vi "Receive Read Data Parse.vi"(8 "error in (no error)":errorcluster, 10 "Specified Num in":u8=1, 11 "Received Read Data":string) -> (0 "error out":errorcluster, 1 "CRC Check?":bool, 2 "Data":i32[](array[numeric]), 3 "Received Read Data":u8[](array[numeric]) format="%.0x")   [LabVIEW 2014, in "ALPHA5 RS485.lvlib"]
uses:
  ALPHA5 RS485.lvlib
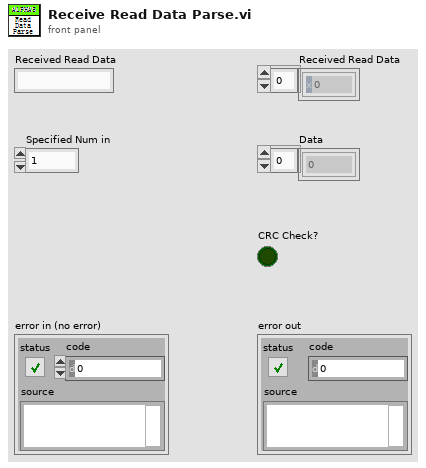
[diagram p1: front panel]
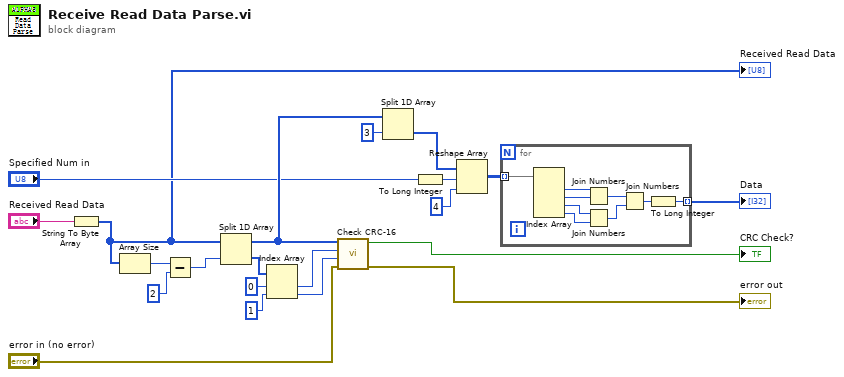
[diagram p0: block diagram]
diagram:
  n1 = String To Byte Array(string="Received Read Data") -> (unsigned byte array=w4:u8[])
  "Received Read Data" <- w4
  n2 = Array Size(array=w4) -> (size(s)=w20:i32)
  n3 = Subtract(x=w20, y=2 ("index")) -> (x-y=w18:i32)
  n4 = Split 1D Array(array=w4, index=w18) -> (first subarray=w12:u8[], second subarray=w17:u8[])
  n5 = Index Array(array=w17, index #1=0 ("index"), index #2=1 ("index")) -> (element #1=w14:u8, element #2=w13:u8)
  n6 = call "Check CRC-16.vi"("error in (no error)"="error in (no error)", "CRC-16-H"=w13, "CRC-16-L"=w14, "Data In"=w12) -> ("error out"=→"error out":errorcluster, "Check Result"=→"CRC Check?":bool)  [unwired: 6 in]
  n7 = Split 1D Array(array=w12, index=3) -> (second subarray=w10:u8[])  [unwired: 1 out]
  n8 = To Long Integer(number="Specified Num in") -> (32bit integer=w9:i32)
  n9 = Reshape Array(w10, w9, 4 ("dimension size")) -> (w7:u8[][])
  n10 = for {
    tunnel: w7 -> [w28] mode=indexing
    tunnel: [w22] -> w6 mode=indexing
    n11 = Index Array(array=w28) -> (element #1=w27:u8, element #2=w26:u8, element #3=w25:u8, element #4=w24:u8)  [unwired: 4 in]
    n12 = Join Numbers(hi=w27, lo=w26) -> ((hi.lo)=w30:u16)
    n13 = Join Numbers(hi=w25, lo=w24) -> ((hi.lo)=w29:u16)
    n14 = Join Numbers(hi=w30, lo=w29) -> ((hi.lo)=w23:u32)
    n15 = To Long Integer(number=w23) -> (32bit integer=w22:i32)
  }
  "Data" <- w6
